vi "calcOD.vi"(10 "channel I":cluster{"BG":sgl[], "Ie":sgl[], "I0":sgl[]}, 11 "channel 2":cluster{"BG":sgl[], "Ie":sgl[], "I0":sgl[]}) -> (1 "Ie":sgl[](array[numeric]), 2 "Ie 2":sgl[](array[numeric]), 3 "OD":sgl[](array[numeric]), 4 "I0 2":sgl[](array[numeric]), 5 "BG":sgl[](array[numeric]), 6 "I0":sgl[](array[numeric]), 7 "BG 2":sgl[](array[numeric]))   [LabVIEW 2020, in "Detector.lvclass"]
uses:
  Detector.lvclass
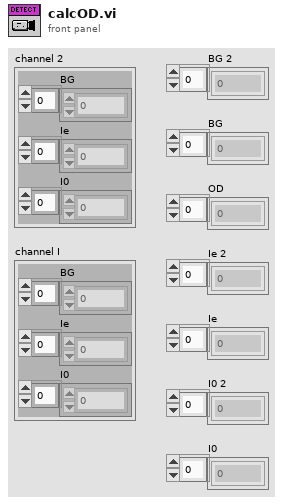
[diagram p1: front panel]
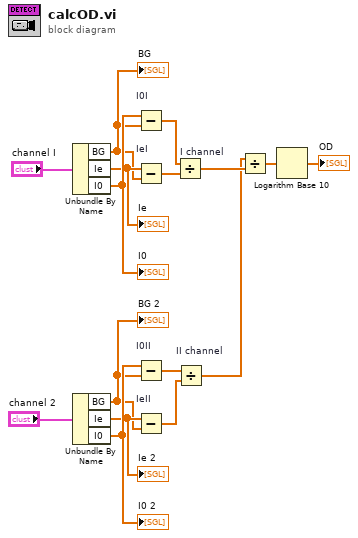
[diagram p0: block diagram]
diagram:
  n1 = Unbundle By Name("channel I") -> ("BG"=w10:sgl[], "Ie"=w13:sgl[], "I0"=w15:sgl[])
  "I0" <- w15
  "Ie" <- w13
  "BG" <- w10
  n2 = Unbundle By Name("channel 2") -> ("BG"=w9:sgl[], "Ie"=w12:sgl[], "I0"=w14:sgl[])
  "I0 2" <- w14
  "Ie 2" <- w12
  "BG 2" <- w9
  n3 = Subtract "I0I"(x=w15, y=w10) -> (x-y=w7:sgl[])
  n4 = Subtract "IeI"(x=w13, y=w10) -> (x-y=w6:sgl[])
  n5 = Subtract "I0II"(x=w14, y=w9) -> (x-y=w8:sgl[])
  n6 = Subtract "IeII"(x=w12, y=w9) -> (x-y=w11:sgl[])
  n7 = Divide "I channel"(x=w7, y=w6) -> (x/y=w5:sgl[])
  n8 = Divide "II channel"(x=w8, y=w11) -> (x/y=w4:sgl[])
  n9 = Divide(x=w4, y=w5) -> (x/y=w3:sgl[])
  n10 = Logarithm Base 10(1:w3) -> (0:→"OD":sgl[])
